vi "getDforce-woutgains.vi"(6 "ForceDesired":dbl, 7 "Desired Direction":dbl[](array[numeric])) -> (3 "FX FY Fz 0 0 0":dbl[](array[numeric]))   [LabVIEW 2017]
uses:
  <vilib>/Analysis/_algsub.llb/Real Vector Norm.vi
  <vilib>/Analysis/NI_AALPro.lvlib
panel:
  out "norm":dbl
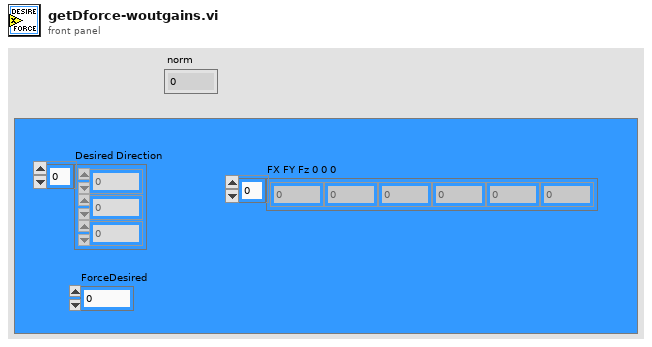
[diagram p1: front panel]
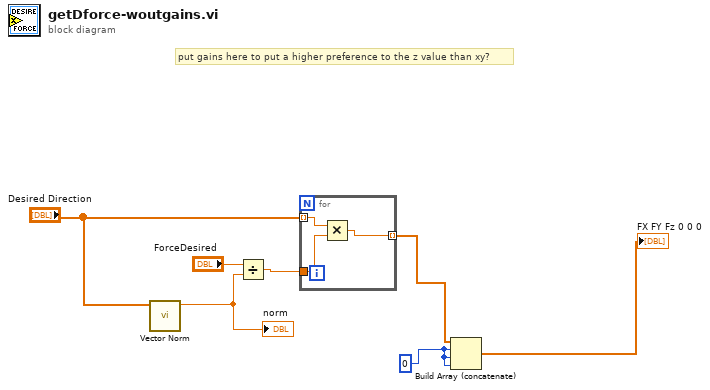
[diagram p0: block diagram]
diagram:
  w2 = 0
  # "put gains here to put a higher preference to the z value than xy?"
  n1 = call-poly <vilib>:"Vector Norm.vi"("Input Vector"="Desired Direction") -> ("norm"=w5:dbl)  [unwired: 9 in, 1 out]
  "norm" <- w5
  n2 = Divide(x="ForceDesired", y=w5) -> (x/y=w7:dbl)
  n3 = for {
    tunnel: "Desired Direction" -> [w10] mode=indexing
    tunnel: w7 -> [w9]
    tunnel: [w8] -> w3 mode=indexing
    n4 = Multiply(x=w10, y=w9) -> (x*y=w8:dbl)
  }
  n5 = Build Array (concatenate)(w3, w2, w2, w2) -> (→"FX FY Fz 0 0 0":dbl[])
